vi "Open File.vi"(8 "error in (no error)":errorcluster, 11 "Spectrum Recorder in":refnum<class "Spectrum Recorder.lvclass">) -> (0 "error out":errorcluster, 3 "Spectrum Recorder out":refnum<class "Spectrum Recorder.lvclass">)   [LabVIEW 2016, in "Spectrum Recorder.lvclass"]
uses:
  Spectrum Recorder.lvclass
  File/Controls/File formats.ctl
  Spectrum Recorder.lvclass/Spectrum Recorder.ctl
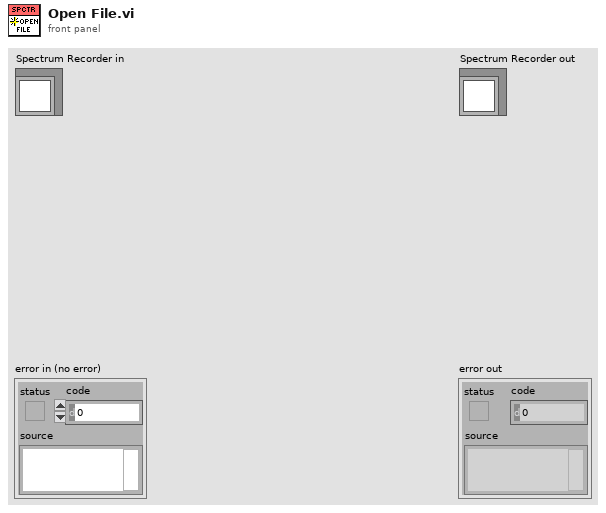
[diagram p1: front panel]
types:
  T1 = enum16{"open", "open or create", "create or replace", "create", "open (read-only)"}
  T2 = typedef "File formats.ctl" = enum16{"TDMS", "ASCII", "BINARY"}
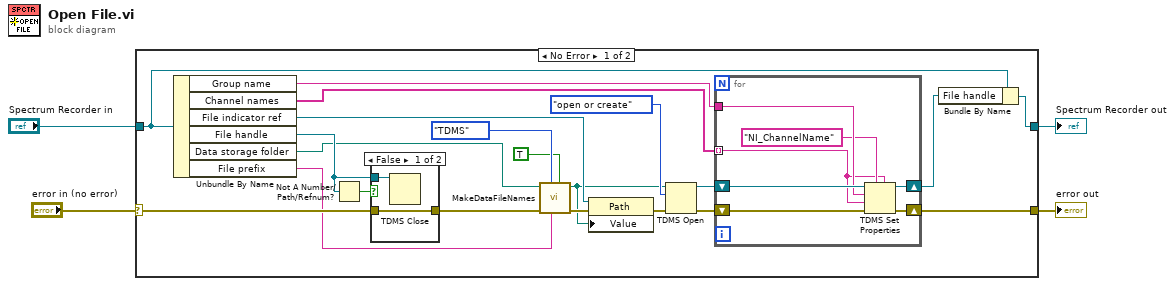
[diagram p0: block diagram]
diagram:
  n1 = case shown="No Error" "error in (no error)" {
    selector: "error in (no error)" -> [w22 w37]
    tunnel: [w5 w37] -> w3
    tunnel: [w15 w36] -> w1
    tunnel: "Spectrum Recorder in" -> [w25 w36]
    frame No Error {
      n2 = Unbundle By Name(w25) -> ("Group name"=w8:string, "Channel names"=w7:string[], "File indicator ref"=w13:refnum<vi>, "File handle"=w23:refnum<k34>, "Data storage folder"=w20:path, "File prefix"=w11:string)
      n3 = Not A Number/Path/Refnum?(number/path/refnum=w23) -> (NaN/Path/Refnum?=w24:bool)
      n4 = case shown="False" w24 {
        tunnel: w23 -> [w34 _]
        tunnel: w22 -> [w33 w35]
        tunnel: [w33 w35] -> w21
        frame False {
          n5 = TDMS Close(11:w34) -> ()  [unwired: 1 in, 2 out]
        }
        frame True {
        }
      }
      n6 = call "MakeDataFileNames.vi"("Include time"=TRUE, "File Prefix"=w11, "File format"=File_formats."TDMS", "Error In"=w21, "Root Data Folder"=w20) -> ("Error Out"=w18:errorcluster, "Data File  Path"=w12:path)  [unwired: 3 in, 2 out]
      n7 = property class="Path"(reference=w13, error in=w18, "Value"=w12) -> (error out=w14:errorcluster)  [unwired: 1 out]
      n8 = TDMS Open(8:w14, 10:T1."open or create" ("operation (0:open)"), 11:w12) -> (0:w6:errorcluster, 3:w10:refnum<k34>)  [unwired: 4 in]
      n9 = for {
        tunnel: w8 -> [w30]
        tunnel: w7 -> [w26] mode=indexing
        shift-right: [w31] -> w9
        shift-left: w10 -> [w32]
        shift-right: [w28] -> w5
        shift-left: w6 -> [w29]
        n10 = TDMS Set Properties(5:w26, 7:"NI_ChannelName", 8:w29, 9:w26, 10:w30, 11:w32) -> (0:w28:errorcluster, 3:w31:refnum<k34>)  [unwired: 2 out]
      }
      n11 = Bundle By Name(cluster=w25, "File handle"=w9) -> (w15:refnum<class "Spectrum Recorder.lvclass">)
    }
    frame Error {
    }
  }
  "error out" <- w3
  "Spectrum Recorder out" <- w1
